vi "data array to waveform.vi"(9 "Main Vari":T1={"Error"={"status"=FALSE, "code"=0, "source"=""}, "Test Info"={"Test Name"="", "Tester"=""}, "StateName"="", "Task Info"={"Accele Task"=[], "Simulate"=FALSE, "采样率"={"AISampleRate"=10123, "CouplingType"=10000, "Butter"=1000}, "Trig"={"PreTrigCNT"=0, "TriggerMode"=enum."中间触发", "TriggerSource"=enum."软件触发", "ATRTriggerChannel"=enum."通道0", "TriggerDir"=enum."下降沿触发", "TrigLevelVolt"=0.0, "bAvailableTrig"=FALSE}, "clock"={"EN"=FALSE, "clocksource"=enum."内部时钟", "outclocksource"=enum."Trig0"}, "delay(S)"=0.0}, "Virb Wave"=[{"t0"=timestamp(3350015091.8292503 s since 1904-01-01), "dt"=0.001, "Y"=array[1000 elements], "attributes"=variant("NI_ChannelName"=variant(string "PXI-6221/ai1"), "NI_UnitDescription"=variant(string "Deg C"))}], "Display Info"=[{"Frequency"=0.0, "RMS"=0.0}, {"Frequency"=0.0, "RMS"=0.0}, {"Frequency"=0.0, "RMS"=0.0}, {"Frequency"=0.0, "RMS"=0.0}, {"Frequency"=0.0, "RMS"=0.0}], "粉尘特性"={"名称"="", "粒径"="", "含水量"=""}, "测试条件"={"初始含氧量"="", "初始压力"="", "测试浓度"="", "点火能量"="", "初始温度"="", "反应器体积[L]"=0.0}, "ch size"=0} {"Task Info"."采样率"."CouplingType" items=["直流耦合", "交流耦合"]}, 11 "data":dbl[](array[numeric])) -> (2 "wave out":waveform(dbl)[](array[waveform]))   [LabVIEW 2011]
uses:
  Ctrls/Main vari.ctl
  Ctrls/Task Info.ctl
  Ctrls/Sample Information.ctl
  Ctrls/Trig.ctl
  Ctrls/clock.ctl
panel:
  in  "set para 2":T10
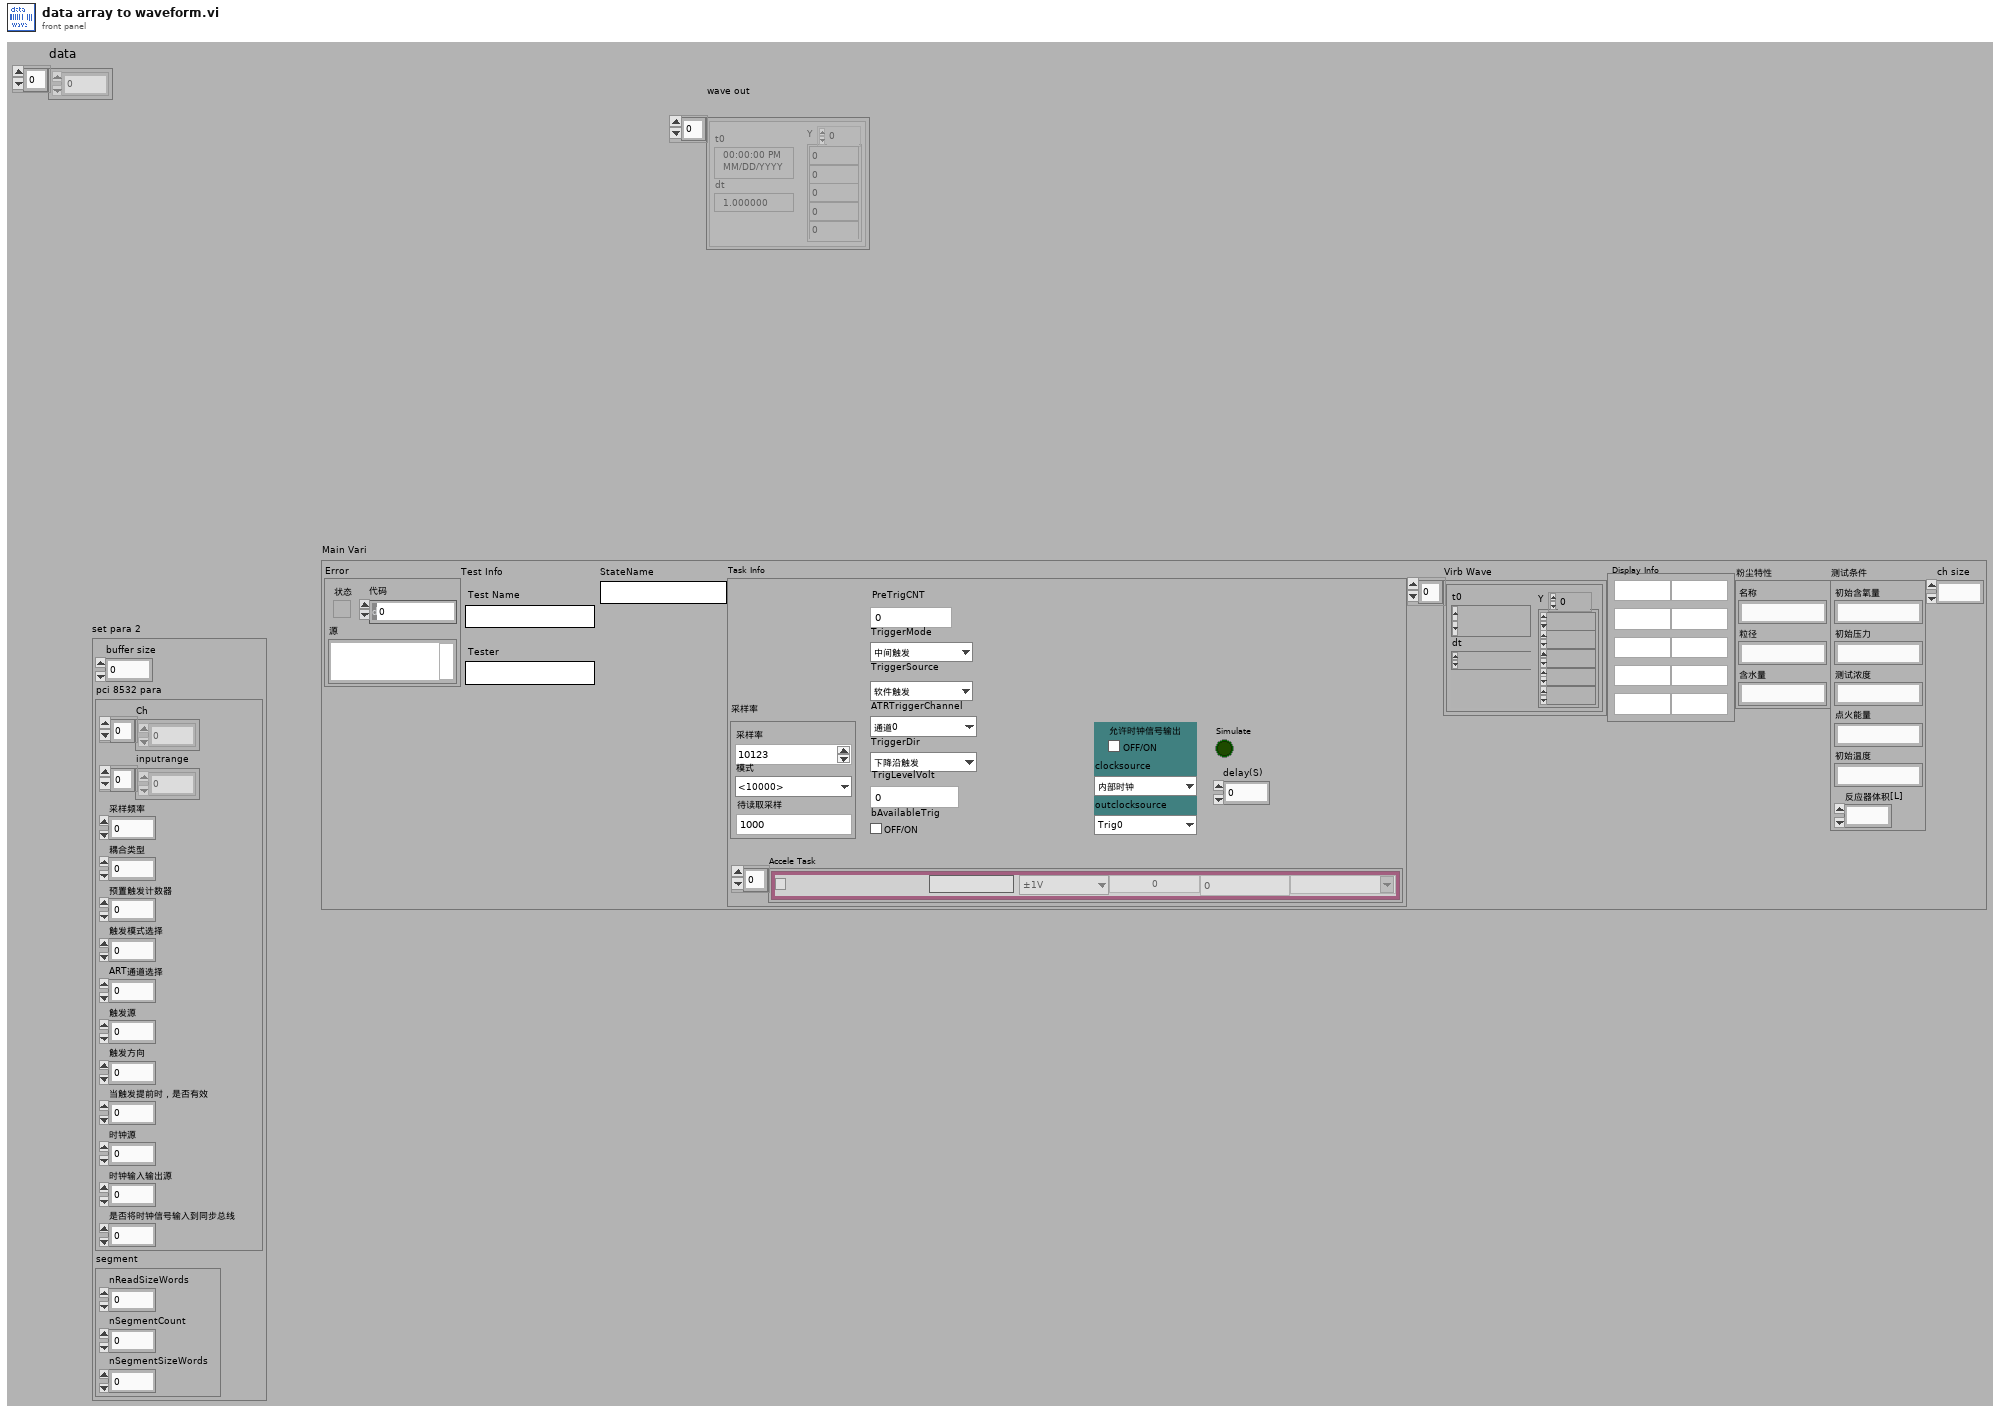
[diagram p1: front panel]
types:
  T1 = typedef "Main vari.ctl" = cluster{"Error":errorcluster, "Test Info":cluster{"Test Name":string, "Tester":string}, "StateName":string, "Task Info":T2, "Virb Wave":waveform(dbl)[], "Display Info":T7, "粉尘特性":T8, "测试条件":T9, "ch size":u8}
  T2 = typedef "Task Info.ctl" = cluster{"Accele Task":T3[], "Simulate":bool, "采样率":T4, "Trig":T5, "clock":T6, "delay(S)":dbl}
  T3 = typedef "Acceleration Channel Config_Ctrls-某型振动实验台测试系统.ctl" = cluster{"Enable":bool, "Name":string, "range":enum16{"±1V", "±5V"}, "SensValue":dbl, "PhysicalName":string, "off":dbl, "Sensunits":string}
  T4 = typedef "Sample Information.ctl" = cluster{"AISampleRate":i32, "CouplingType":i32, "Butter":i32}
  T5 = typedef "Trig.ctl" = cluster{"PreTrigCNT":i32, "TriggerMode":enum16{"中间触发", "后触发", "预触发", "硬件延时触发"}, "TriggerSource":enum16{"软件触发", "DTR信号源", "ATR信号源", "Triger信号触发"}, "ATRTriggerChannel":enum16{"通道0", "通道1", "通道2", "通道3"}, "TriggerDir":enum16{"下降沿触发", "上升沿触发", "上下边没均触发"}, "TrigLevelVolt":sgl, "bAvailableTrig":bool}
  T6 = typedef "clock.ctl" = cluster{"EN":bool, "clocksource":enum16{"内部时钟", "外部时钟"}, "outclocksource":enum16{"Trig0", "Trig1", "Trig2", "Trig3", "Trig4", "Trig5", "Trig6", "Trig7", "PXI_STAR"}}
  T7 = typedef "Display Information_Ctrls-某型振动实验台测试系统.ctl" = cluster{"Frequency":dbl, "RMS":dbl}[]
  T8 = typedef "粉尘特性.ctl" = cluster{"名称":string, "粒径":string, "含水量":string}
  T9 = typedef "测试条件.ctl" = cluster{"初始含氧量":string, "初始压力":string, "测试浓度":string, "点火能量":string, "初始温度":string, "反应器体积[L]":dbl}
  T10 = cluster{"buffer size":i32, "pci 8532 para":cluster{"Ch":i32[], "inputrange":i32[], "采样频率":i32, "耦合类型":i32, "预置触发计数器":i32, "触发模式选择":i32, "ART通道选择":i32, "触发源":i32, "触发方向":i32, "当触发提前时，是否有效":i32, "时钟源":i32, "时钟输入输出源":i32, "是否将时钟信号输入到同步总线":i32}, "segment":cluster{"nReadSizeWords":i32, "nSegmentCount":i32, "nSegmentSizeWords":i32}}
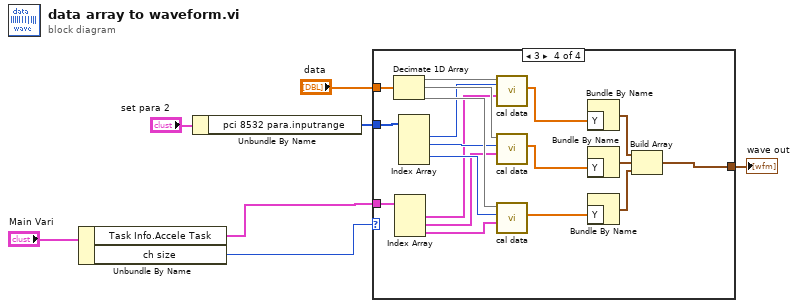
[diagram p0: block diagram]
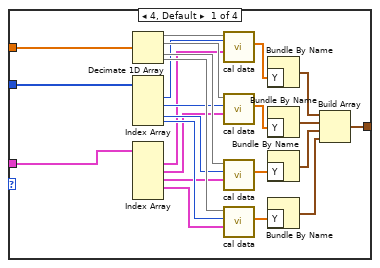
[diagram p2: hidden frame]
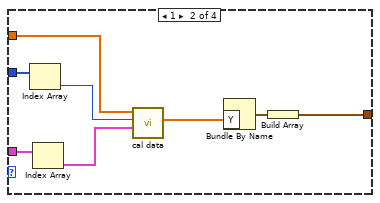
[diagram p3: hidden frame]
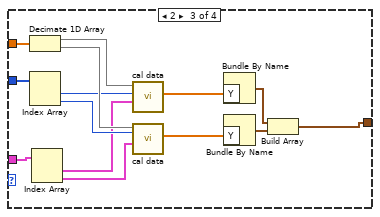
[diagram p4: hidden frame]
diagram:
  n1 = Unbundle By Name("Main Vari") -> ("Task Info.Accele Task"=w1:T3[], "ch size"=w2:u8)
  n2 = Unbundle By Name("set para 2") -> ("pci 8532 para.inputrange"=w5:i32[])
  n3 = case shown="3" w2 {
    tunnel: "data" -> [w31 w32 w53 w72]
    tunnel: w5 -> [w30 w39 w52 w71]
    tunnel: [w13 w35 w43 w58] -> w4
    tunnel: w1 -> [w8 w33 w40 w54]
    frame 4, Default {
      n4 = Decimate 1D Array(w31) -> (w29:dbl[], w28:dbl[], w27:dbl[], w26:dbl[])
      n5 = Index Array(array=w30) -> (element #1=w25:i32, element #2=w24:i32, element #3=w23:i32, element #4=w22:i32)  [unwired: 4 in]
      n6 = Index Array(array=w8) -> (element #1=w12:T3, element #2=w11:T3, element #3=w10:T3, element #4=w9:T3)  [unwired: 5 in, 1 out]
      n7 = call "cal data.vi"("输入簇"=w12, "range"=w25, "data"=w29) -> ("data out"=w21:dbl[])  [unwired: 8 out]
      n8 = call "cal data.vi"("输入簇"=w11, "range"=w24, "data"=w28) -> ("data out"=w20:dbl[])  [unwired: 8 out]
      n9 = call "cal data.vi"("输入簇"=w10, "range"=w23, "data"=w27) -> ("data out"=w19:dbl[])  [unwired: 8 out]
      n10 = call "cal data.vi"("输入簇"=w9, "range"=w22, "data"=w26) -> ("data out"=w18:dbl[])  [unwired: 8 out]
      n11 = Bundle By Name("Y"=w21) -> (w17:waveform(dbl))  [unwired: 1 in]
      n12 = Bundle By Name("Y"=w20) -> (w16:waveform(dbl))  [unwired: 1 in]
      n13 = Bundle By Name("Y"=w19) -> (w15:waveform(dbl))  [unwired: 1 in]
      n14 = Bundle By Name("Y"=w18) -> (w14:waveform(dbl))  [unwired: 1 in]
      n15 = Build Array(w17, w16, w15, w14) -> (w13:waveform(dbl)[])
    }
    frame 1 {
      n16 = Index Array(array=w39) -> (element=w38:i32)  [unwired: 1 in]
      n17 = Index Array(array=w33) -> (element=w34:T3)  [unwired: 1 in]
      n18 = call "cal data.vi"("输入簇"=w34, "range"=w38, "data"=w32) -> ("data out"=w37:dbl[])  [unwired: 8 out]
      n19 = Bundle By Name("Y"=w37) -> (w36:waveform(dbl))  [unwired: 1 in]
      n20 = Build Array(w36) -> (w35:waveform(dbl)[])
    }
    frame 2 {
      n21 = Decimate 1D Array(w53) -> (w51:dbl[], w50:dbl[])
      n22 = Index Array(array=w52) -> (element #1=w49:i32, element #2=w48:i32)  [unwired: 2 in]
      n23 = Index Array(array=w40) -> (element #1=w42:T3, element #2=w41:T3)  [unwired: 2 in]
      n24 = call "cal data.vi"("输入簇"=w42, "range"=w49, "data"=w51) -> ("data out"=w47:dbl[])  [unwired: 8 out]
      n25 = call "cal data.vi"("输入簇"=w41, "range"=w48, "data"=w50) -> ("data out"=w46:dbl[])  [unwired: 8 out]
      n26 = Bundle By Name("Y"=w47) -> (w45:waveform(dbl))  [unwired: 1 in]
      n27 = Bundle By Name("Y"=w46) -> (w44:waveform(dbl))  [unwired: 1 in]
      n28 = Build Array(w45, w44) -> (w43:waveform(dbl)[])
    }
    frame 3 {
      n29 = Decimate 1D Array(w72) -> (w70:dbl[], w69:dbl[], w68:dbl[])
      n30 = Index Array(array=w54) -> (element #1=w57:T3, element #2=w56:T3, element #3=w55:T3)  [unwired: 3 in]
      n31 = Index Array(array=w71) -> (element #1=w67:i32, element #2=w66:i32, element #3=w65:i32)  [unwired: 4 in, 1 out]
      n32 = call "cal data.vi"("输入簇"=w57, "range"=w67, "data"=w70) -> ("data out"=w64:dbl[])  [unwired: 8 out]
      n33 = call "cal data.vi"("输入簇"=w56, "range"=w66, "data"=w69) -> ("data out"=w63:dbl[])  [unwired: 8 out]
      n34 = call "cal data.vi"("输入簇"=w55, "range"=w65, "data"=w68) -> ("data out"=w62:dbl[])  [unwired: 8 out]
      n35 = Bundle By Name("Y"=w64) -> (w61:waveform(dbl))  [unwired: 1 in]
      n36 = Bundle By Name("Y"=w63) -> (w60:waveform(dbl))  [unwired: 1 in]
      n37 = Bundle By Name("Y"=w62) -> (w59:waveform(dbl))  [unwired: 1 in]
      n38 = Build Array(w61, w60, w59) -> (w58:waveform(dbl)[])
    }
  }
  "wave out" <- w4
